vi "test_advanced_Doppler.vi"() -> ()   [LabVIEW 2009]
doc: "Copyright (C) 2009, Stepan A. Baranov\nweb: http://www.OCTLab.org/\nemail: stepan@baranov.su"
uses:
  OCTLib.dll
panel:
  out "version":string
  out "name":string
  out "error out":errorcluster
  out "cell height":i32
  out "cell width":i32
  out "A-scan size":i32
  out "# of A-scans":i32
  in  "Small/Big":bool
  out "loop #":i32
  out "RSM_STAT time":u32
  out "LabView time":u32
  out "RSM_STAT Array":dbl[][](array[numeric])
  out "LabView Array":dbl[][](array[numeric])
  in  "stop":bool
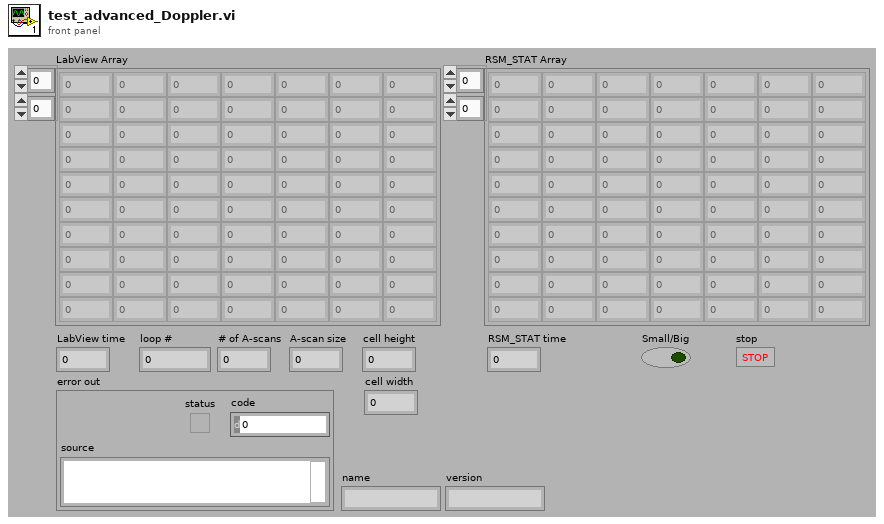
[diagram p1: front panel]
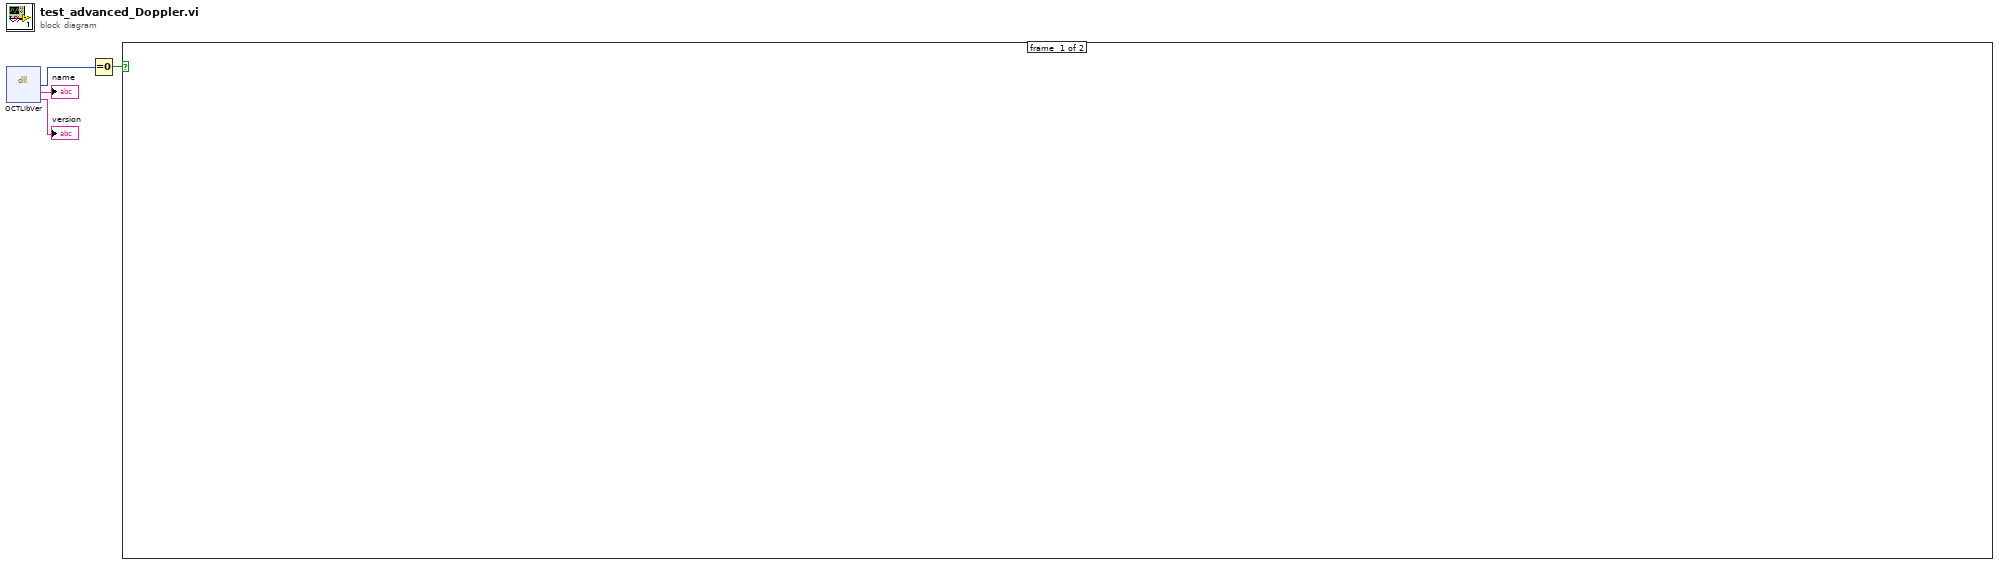
[diagram p0: block diagram]
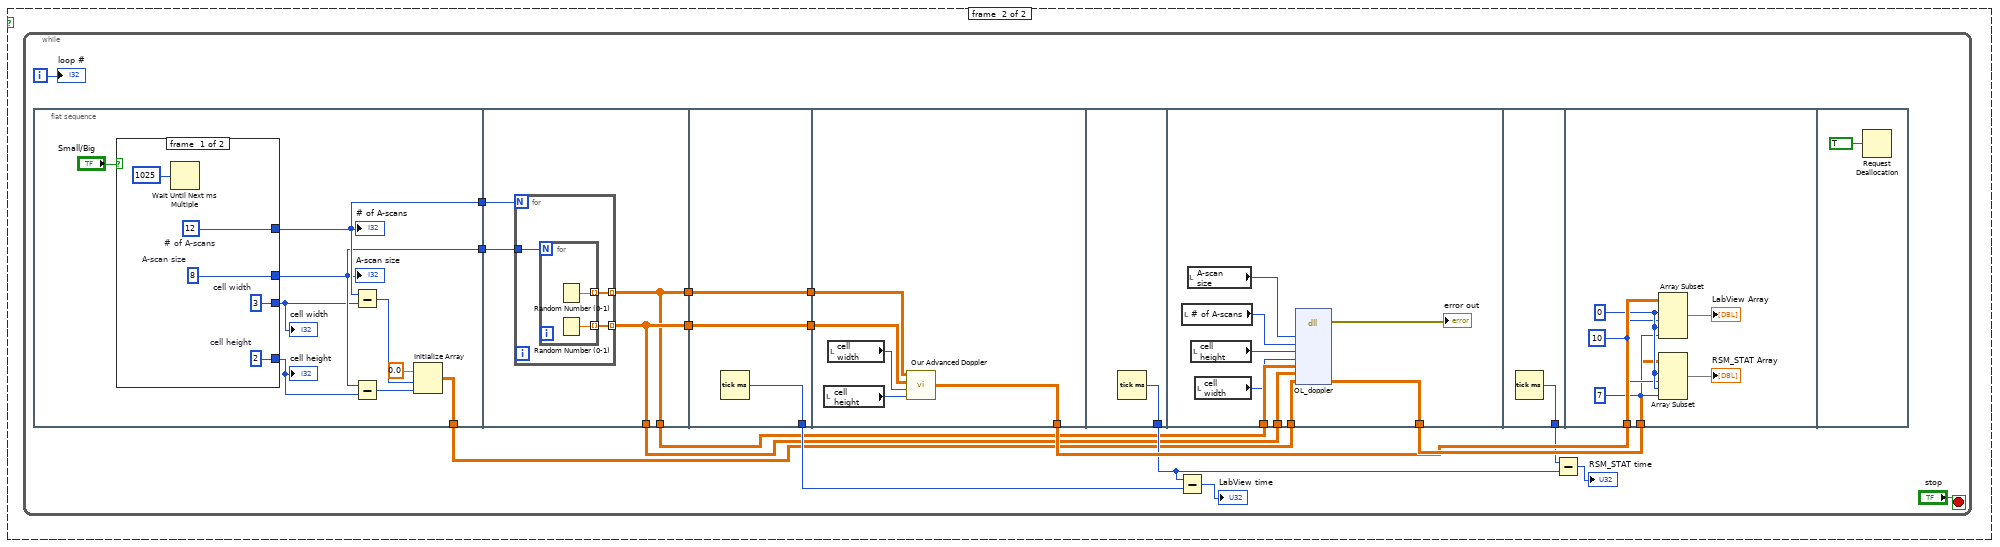
[diagram p2: hidden frame]
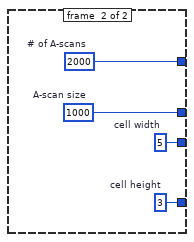
[diagram p3: hidden frame]
diagram:
  n1 = dll-call lib="OCTLib.dll" fn="OCTLibVer"() -> ("status"=w4:i8, "name"=→"name":string, "version"=→"version":string)  [unwired: 5 in, 2 out]
  n2 = Equal To 0?(x=w4) -> (x = 0?=w3:bool)
  n3 = case shown="True" w3 {
    frame #0 {
    }
    frame #1 {
      n4 = while {
        i -> [w14]
        stop <- "stop" stop-if-true
        n5 = flat-sequence {
          tunnel: [w27] -> w10
          tunnel: [w30] -> w9
          tunnel: [w25] -> w5
          tunnel: [w42] -> w13
          tunnel: [w42] -> w11
          tunnel: w10 -> [w44]
          tunnel: w9 -> [w43]
          tunnel: [w41] -> w8
          tunnel: [w41] -> w6
          tunnel: [w52] -> w19
          tunnel: [w51] -> w12
          tunnel: w11 -> [w51]
          tunnel: w8 -> [w50]
          tunnel: [w50] -> w7
          tunnel: [w55] -> w20
          tunnel: w12 -> [w56]
          tunnel: w7 -> [w57]
          tunnel: [w58] -> w16
          tunnel: w13 -> [w64]
          tunnel: [w67] -> w21
          tunnel: w6 -> [w63]
          tunnel: w5 -> [w60]
          tunnel: [w68] -> w17
          tunnel: w21 -> [w69]
          tunnel: w20 -> [w75]
          frame #0 {
            n6 = case shown="False" "Small/Big" {
              tunnel: [w35 w39] -> w30
              tunnel: [w36 w40] -> w27
              tunnel: [w33 w38] -> w23
              tunnel: [w32 w37] -> w24
              frame #0 {
                w32 = 2  # cell height
                w33 = 3  # cell width
                w36 = 8  # A-scan size
                w35 = 12  # # of A-scans
                n7 = Wait Until Next ms Multiple(millisecond multiple=u32 1025) -> ()  [unwired: 1 out]
              }
              frame #1 {
                w37 = 3  # cell height
                w38 = 5  # cell width
                w40 = 1000  # A-scan size
                w39 = 2000  # # of A-scans
              }
            }
            "# of A-scans" <- w30
            "A-scan size" <- w27
            "cell width" <- w23
            "cell height" <- w24
            n8 = Subtract(x=w30, y=w23) -> (x-y=w29:i32)
            n9 = Subtract(x=w27, y=w24) -> (x-y=w26:i32)
            n10 = Initialize Array(0.0 ("element"), w29, w26) -> (w25:dbl[][])
          }
          frame #1 {
            n11 = for {
              N: w43 -> [_]
              tunnel: w44 -> [w47]
              tunnel: [w46] -> w42 mode=indexing
              tunnel: [w45] -> w41 mode=indexing
              n12 = for {
                N: w47 -> [_]
                tunnel: [w49] -> w46 mode=indexing
                tunnel: [w48] -> w45 mode=indexing
                n13 = Random Number (0-1)() -> (number: 0 to 1=w48:dbl)
                n14 = Random Number (0-1)() -> (number: 0 to 1=w49:dbl)
              }
            }
          }
          frame #2 {
            n15 = Tick Count (ms)() -> (millisecond timer value=w52:u32)
          }
          frame #3 {
            n16 = local read "cell height"() -> (w53:i32)
            n17 = local read "cell width"() -> (w54:i32)
            n18 = call "Our Advanced Doppler.vi"("cell height"=w53, "cell width"=w54, "Imaginary Part"=w56, "Real Part"=w57) -> ("2D Doppler Image"=w55:dbl[][])
          }
          frame #4 {
            n19 = Tick Count (ms)() -> (millisecond timer value=w58:u32)
          }
          frame #5 {
            n20 = local read "# of A-scans"() -> (w65:i32)
            n21 = local read "A-scan size"() -> (w66:i32)
            n22 = local read "cell height"() -> (w62:i32)
            n23 = local read "cell width"() -> (w61:i32)
            n24 = dll-call lib="OCTLib.dll" fn="OL_doppler"("A-scan size"=w66, "# of A-scan"=w65, "cell height"=w62, "cell width"=w61, "Re"=w63, "Im"=w64, "data"=w60) -> (error out=→"error out":errorcluster, "data"=w67:dbl[][])  [unwired: 10 in, 1 out]
          }
          frame #6 {
            n25 = Tick Count (ms)() -> (millisecond timer value=w68:u32)
          }
          frame #7 {
            w72 = 10 ("length")
            w71 = 7 ("length")
            w73 = 0 ("index")
            n26 = Array Subset(array=w75, index (row)=w73, length (row)=w72, index (col)=w73, length (col)=w71) -> (→"LabView Array":dbl[][])
            n27 = Array Subset(array=w69, index (row)=w73, length (row)=w72, index (col)=w73, length (col)=w71) -> (→"RSM_STAT Array":dbl[][])
          }
          frame #8 {
            n28 = Request Deallocation(TRUE ("flag")) -> ()
          }
        }
        n29 = Subtract(x=w16, y=w19) -> (x-y=→"LabView time":u32)
        n30 = Subtract(x=w17, y=w16) -> (x-y=→"RSM_STAT time":u32)
        "loop #" <- w14
      }
    }
  }
